vi "Command_Joint_Angles_cluster.vi"(4 "Mode":enum16{"Position", "Velocity", "Effort"}(ring), 5 "node":string, 6 "error in":errorcluster, 7 "Arm Angles (degrees)":T1, 9 "Side":T2) -> (0 "error out":errorcluster)   [LabVIEW 2013]
uses:
  ROS/Code/SubVIs/BaxterSide.ctl
  ROS/Code/SubVIs/BaxterArmsSmall.ctl
panel:
  out "Move Command":string
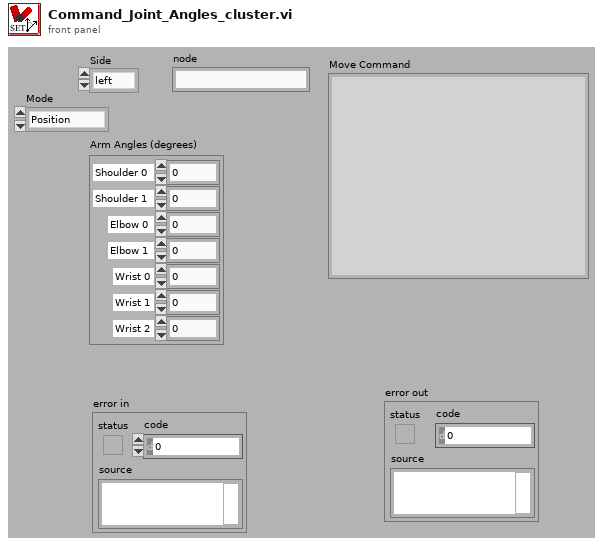
[diagram p1: front panel]
types:
  T1 = typedef "BaxterArmsSmall.ctl" = cluster{"Elbow 0":dbl, "Elbow 1":dbl, "Shoulder 0":dbl, "Shoulder 1":dbl, "Wrist 0":dbl, "Wrist 1":dbl, "Wrist 2":dbl}
  T2 = typedef "BaxterSide.ctl" = enum16{"left", "right"}
  T3 = typedef "_ROSControl.ctl" = cluster{"topic port":u16, "Node":string, "topic":string, "type":string, "node port":u32, "error ":errorcluster, "Direction":T4, "APIs":string[]}
  T4 = typedef "_ROSDirection.ctl" = enum16{"Node", "Publisher", "Subscriber", "Service Client"}
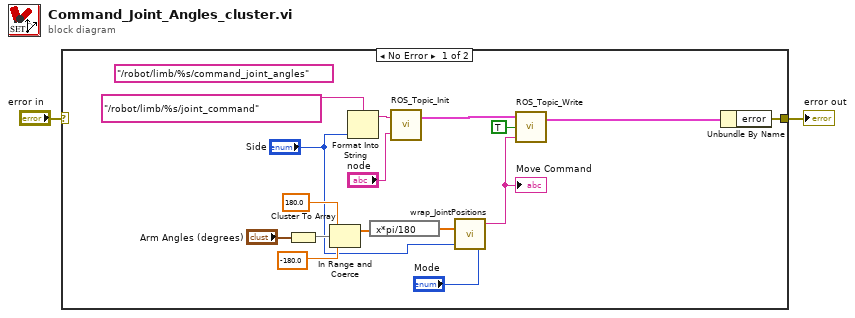
[diagram p0: block diagram]
diagram:
  n1 = case shown="No Error" "error in" {
    selector: "error in" -> [_ w19]
    tunnel: [w18 w19] -> w2
    frame No Error {
      (unwired) "/robot/limb/%s/command_joint_angles" ("topic")
      n2 = Cluster To Array(cluster="Arm Angles (degrees)") -> (array=w12:dbl[])
      n3 = In Range and Coerce(upper limit=180.0 ("Elbow 0"), x=w12, lower limit=-180.0 ("Elbow 0")) -> (coerced(x)=w8:dbl[])  [unwired: 1 out]
      n4 = Format Into String(format string="/robot/limb/%s/joint_command" ("topic"), "Side") -> (resulting string=w16:string)  [unwired: 2 in, 1 out]
      n5 = expression code="x*pi/180"(w8) -> (w7:dbl[])
      n6 = call "ROS_Topic_Init.vi"("node"="node", "topic"=w16) -> ("ROS out"=w15:T3)  [unwired: 1 in]
      n7 = call "wrap_JointPositions.vi"("Mode"="Mode", "Side"="Side", "Positions"=w7) -> ("msg out"=w9:string)  [unwired: 2 in]
      "Move Command" <- w9
      n8 = call "ROS_Topic_Write.vi"("Msg in"=w9, "Continuous?"=TRUE, "ROS in"=w15) -> ("ROS out"=w14:T3)  [unwired: 1 in]
      n9 = Unbundle By Name(w14) -> ("error"=w18:errorcluster)
    }
    frame Error {
    }
  }
  "error out" <- w2
